vi "Visible_Ch.vi"(8 "Unit PN":string) -> ()   [LabVIEW 2017]
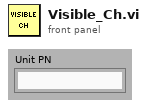
[diagram p1: front panel]
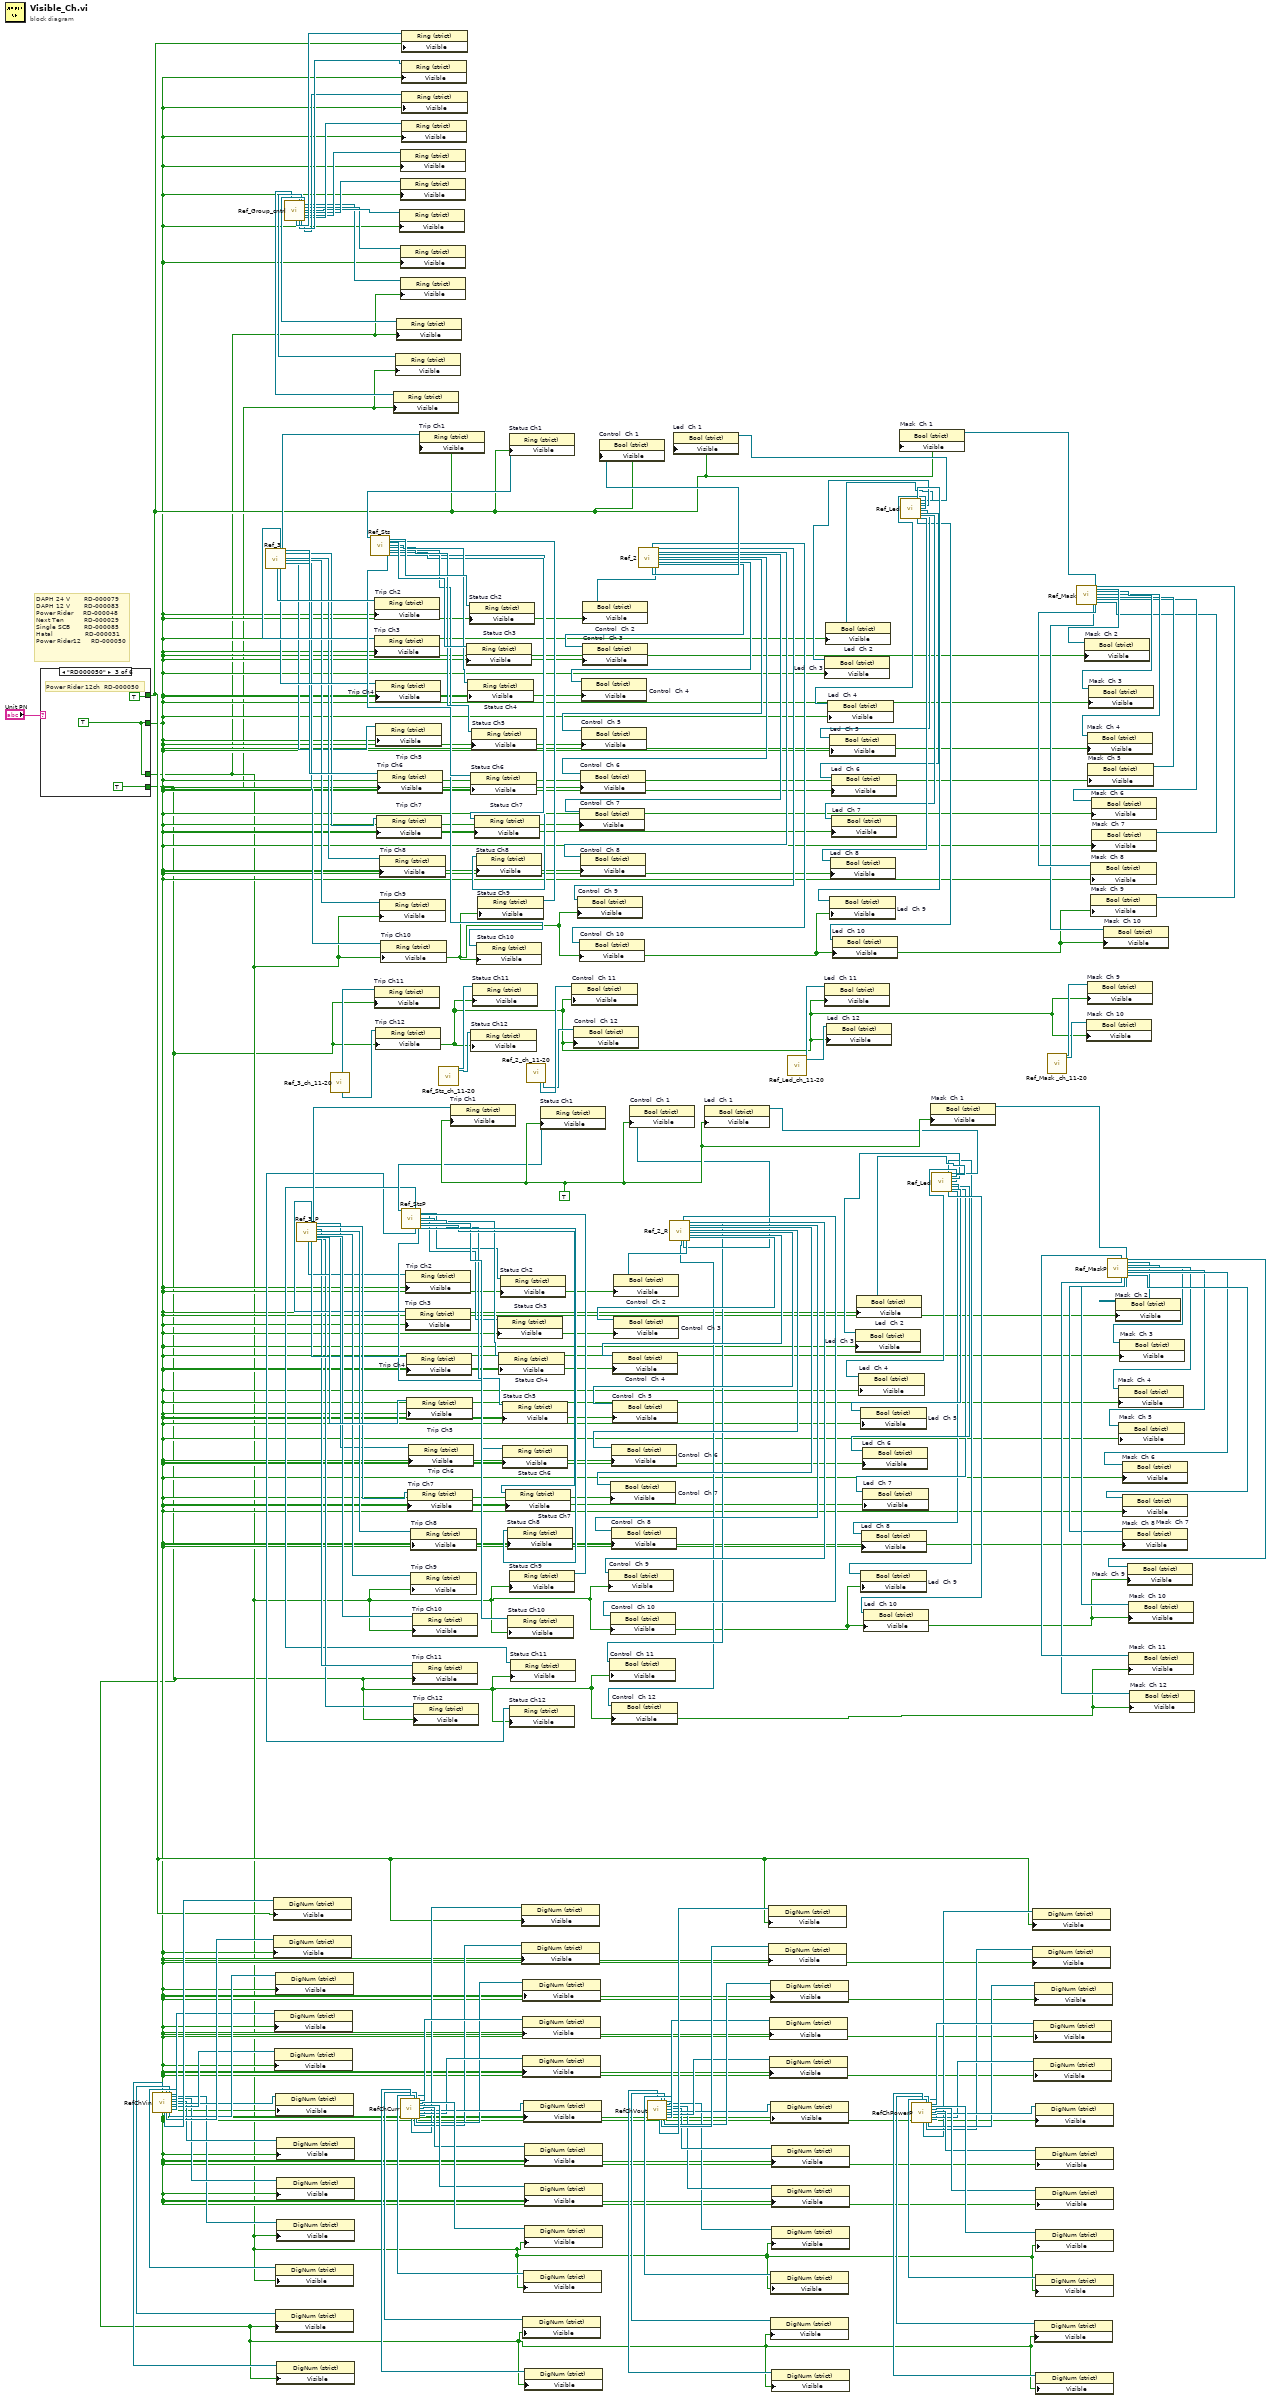
[diagram p0: block diagram]
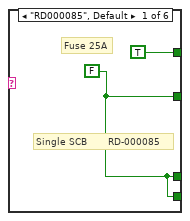
[diagram p2: hidden frame]
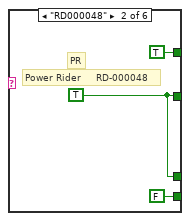
[diagram p3: hidden frame]
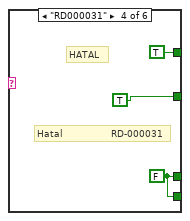
[diagram p4: hidden frame]
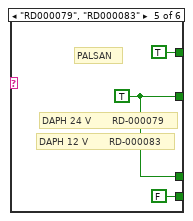
[diagram p5: hidden frame]
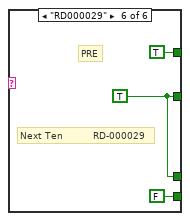
[diagram p6: hidden frame]
diagram:
  w133 = TRUE
  # "DAPH 24 V  \t    RD-000079\nDAPH 12 V  \t    RD-000083\nPower Rider \t   RD-000048\nNext Ten  \t       RD-000029\nSingle SCB       RD-000085 \nHatal                RD-000031\nPower Rider12 \t   RD-000050"
  n1 = case shown="\"RD000050\"" "Unit PN" {
    tunnel: [w186 w189 w192 TRUE w198 w201] -> w3
    tunnel: [w186 w189 w192 w194 w198 w201] -> w2
    tunnel: [w186 FALSE TRUE w194 FALSE FALSE] -> w1
    tunnel: [TRUE TRUE TRUE TRUE TRUE TRUE] -> w4
    frame "RD000085", Default {
      w186 = FALSE
      # "Single SCB       RD-000085"
      # "Fuse 25A"
    }
    frame "RD000048" {
      w189 = TRUE
      # "Power Rider \t   RD-000048"
      # "PR"
    }
    frame "RD000050" {
      w192 = TRUE
      # "Power Rider 12ch  RD-000050"
    }
    frame "RD000031" {
      w194 = FALSE
      # "Hatal                RD-000031"
      # "HATAL"
    }
    frame "RD000079", "RD000083" {
      w198 = TRUE
      # "DAPH 12 V  \t    RD-000083"
      # "DAPH 24 V  \t    RD-000079"
      # "PALSAN"
    }
    frame "RD000029" {
      w201 = TRUE
      # "Next Ten  \t       RD-000029"
      # "PRE"
    }
  }
  n2 = call "RefChVin.vi"() -> ("Vin  P1 out"=w64:refnum<vi>, "Vin  P12 out"=w53:refnum<vi>, "Vin  P2 out"=w63:refnum<vi>, "Vin  P11 out"=w54:refnum<vi>, "Vin  P3 out"=w62:refnum<vi>, "Vin  P10 out"=w55:refnum<vi>, "Vin  P9 out"=w56:refnum<vi>, "Vin  P8 out"=w57:refnum<vi>, "Vin  P7 out"=w58:refnum<vi>, "Vin  P6 out"=w59:refnum<vi>, "Vin  P5 out"=w60:refnum<vi>, "Vin  P4 out"=w61:refnum<vi>)  [unwired: 15 in, 1 out]
  n3 = call "Ref_3.vi"() -> ("Trip  Ch 1 out"=w184:refnum<vi>, "Trip  Ch 2 out"=w180:refnum<vi>, "Trip  Ch 3 out"=w164:refnum<vi>, "Trip  Ch 4 out"=w163:refnum<vi>, "Trip  Ch 5 out"=w144:refnum<vi>, "Trip  Ch 6 out"=w162:refnum<vi>, "Trip  Ch 7 out"=w161:refnum<vi>, "Trip  Ch 8 out"=w160:refnum<vi>, "Trip  Ch 9 out"=w159:refnum<vi>, "Trip  Ch 10 out"=w158:refnum<vi>)  [unwired: 18 in]
  n4 = property class="DigNum (strict)"(reference=w64, "Visible"=w4) -> ()  [unwired: 1 in, 2 out]
  n5 = property class="DigNum (strict)"(reference=w63, "Visible"=w3) -> ()  [unwired: 1 in, 2 out]
  n6 = property class="DigNum (strict)"(reference=w61, "Visible"=w3) -> ()  [unwired: 1 in, 2 out]
  n7 = property class="DigNum (strict)"(reference=w60, "Visible"=w3) -> ()  [unwired: 1 in, 2 out]
  n8 = property class="DigNum (strict)"(reference=w62, "Visible"=w3) -> ()  [unwired: 1 in, 2 out]
  n9 = property class="DigNum (strict)"(reference=w54, "Visible"=w1) -> ()  [unwired: 1 in, 2 out]
  n10 = property class="DigNum (strict)"(reference=w59, "Visible"=w3) -> ()  [unwired: 1 in, 2 out]
  n11 = property class="DigNum (strict)"(reference=w55, "Visible"=w2) -> ()  [unwired: 1 in, 2 out]
  n12 = property class="DigNum (strict)"(reference=w58, "Visible"=w3) -> ()  [unwired: 1 in, 2 out]
  n13 = property class="DigNum (strict)"(reference=w57, "Visible"=w3) -> ()  [unwired: 1 in, 2 out]
  n14 = property class="DigNum (strict)"(reference=w56, "Visible"=w2) -> ()  [unwired: 1 in, 2 out]
  n15 = property class="DigNum (strict)"(reference=w53, "Visible"=w1) -> ()  [unwired: 1 in, 2 out]
  n16 = call "Ref_Group_cntrl.vi"() -> ("Group ch 1 out"=w16:refnum<vi>, "Group ch 12 out"=w5:refnum<vi>, "Group ch 2 out"=w15:refnum<vi>, "Group ch 11 out"=w6:refnum<vi>, "Group ch 3 out"=w14:refnum<vi>, "Group ch 10 out"=w7:refnum<vi>, "Group ch 9 out"=w8:refnum<vi>, "Group ch 8 out"=w9:refnum<vi>, "Group ch 7 out"=w10:refnum<vi>, "Group ch 6 out"=w11:refnum<vi>, "Group ch 5 out"=w12:refnum<vi>, "Group ch 4 out"=w13:refnum<vi>)  [unwired: 15 in, 1 out]
  n17 = call "Ref_3_P.vi"() -> ("Trip  Ch 1 out"=w83:refnum<vi>, "Trip  Ch 2 out"=w86:refnum<vi>, "Trip  Ch 3 out"=w102:refnum<vi>, "Trip  Ch 4 out"=w103:refnum<vi>, "Trip  Ch 5 out"=w122:refnum<vi>, "Trip  Ch 6 out"=w104:refnum<vi>, "Trip  Ch 7 out"=w105:refnum<vi>, "Trip  Ch 11 out"=w82:refnum<vi>, "Trip  Ch 8 out"=w106:refnum<vi>, "Trip  Ch 9 out"=w107:refnum<vi>, "Trip  Ch 10 out"=w108:refnum<vi>, "Trip  Ch 12 out"=w81:refnum<vi>)  [unwired: 16 in]
  n18 = call "Ref_3_ch_11-20.vi"() -> ("Trip  Ch 11 out"=w68:refnum<vi>, "Trip  Ch 12 out"=w67:refnum<vi>)  [unwired: 18 in, 8 out]
  n19 = call "Ref_Sts.vi"() -> ("Status Ch9 out"=w166:refnum<vi>, "Status Ch10 out"=w165:refnum<vi>, "Status Ch1 out"=w183:refnum<vi>, "Status Ch2 out"=w172:refnum<vi>, "Status Ch3 out"=w171:refnum<vi>, "Status Ch4 out"=w170:refnum<vi>, "Status Ch5 out"=w169:refnum<vi>, "Status Ch6 out"=w168:refnum<vi>, "Status Ch7 out"=w167:refnum<vi>, "Status Ch8 out"=w155:refnum<vi>)  [unwired: 18 in]
  n20 = property on="Trip Ch3" class="Ring (strict)"(reference=w164, "Visible"=w3) -> ()  [unwired: 1 in, 2 out]
  n21 = property on="Trip Ch11" class="Ring (strict)"(reference=w68, "Visible"=w1) -> ()  [unwired: 1 in, 2 out]
  n22 = property on="Trip Ch2" class="Ring (strict)"(reference=w180, "Visible"=w3) -> ()  [unwired: 1 in, 2 out]
  n23 = property on="Trip Ch4" class="Ring (strict)"(reference=w163, "Visible"=w3) -> ()  [unwired: 1 in, 2 out]
  n24 = property on="Trip Ch12" class="Ring (strict)"(reference=w67, "Visible"=w1) -> ()  [unwired: 1 in, 2 out]
  n25 = property on="Trip Ch5" class="Ring (strict)"(reference=w144, "Visible"=w3) -> ()  [unwired: 1 in, 2 out]
  n26 = property on="Trip Ch7" class="Ring (strict)"(reference=w161, "Visible"=w3) -> ()  [unwired: 1 in, 2 out]
  n27 = property on="Trip Ch6" class="Ring (strict)"(reference=w162, "Visible"=w3) -> ()  [unwired: 1 in, 2 out]
  n28 = property on="Trip Ch8" class="Ring (strict)"(reference=w160, "Visible"=w3) -> ()  [unwired: 1 in, 2 out]
  n29 = property on="Trip Ch9" class="Ring (strict)"(reference=w159, "Visible"=w2) -> ()  [unwired: 1 in, 2 out]
  n30 = property on="Trip Ch10" class="Ring (strict)"(reference=w158, "Visible"=w2) -> ()  [unwired: 1 in, 2 out]
  n31 = property class="Ring (strict)"(reference=w5, "Visible"=w1) -> ()  [unwired: 1 in, 2 out]
  n32 = property class="Ring (strict)"(reference=w6, "Visible"=w1) -> ()  [unwired: 1 in, 2 out]
  n33 = property class="Ring (strict)"(reference=w7, "Visible"=w2) -> ()  [unwired: 1 in, 2 out]
  n34 = property class="Ring (strict)"(reference=w10, "Visible"=w3) -> ()  [unwired: 1 in, 2 out]
  n35 = property class="Ring (strict)"(reference=w12, "Visible"=w3) -> ()  [unwired: 1 in, 2 out]
  n36 = property class="Ring (strict)"(reference=w11, "Visible"=w3) -> ()  [unwired: 1 in, 2 out]
  n37 = property class="Ring (strict)"(reference=w9, "Visible"=w3) -> ()  [unwired: 1 in, 2 out]
  n38 = call "RefChCurr.vi"() -> ("Current P1 out"=w41:refnum<vi>, "Current P12 out"=w52:refnum<vi>, "Current P2 out"=w42:refnum<vi>, "Current P11 out"=w51:refnum<vi>, "Current P3 out"=w43:refnum<vi>, "Current P10 out"=w50:refnum<vi>, "Current P9 out"=w49:refnum<vi>, "Current P8 out"=w48:refnum<vi>, "Current P7 out"=w47:refnum<vi>, "Current P6 out"=w46:refnum<vi>, "Current P5 out"=w45:refnum<vi>, "Current P4 out"=w44:refnum<vi>)  [unwired: 15 in, 1 out]
  n39 = property class="Ring (strict)"(reference=w8, "Visible"=w2) -> ()  [unwired: 1 in, 2 out]
  n40 = property class="Ring (strict)"(reference=w15, "Visible"=w3) -> ()  [unwired: 1 in, 2 out]
  n41 = property class="Ring (strict)"(reference=w13, "Visible"=w3) -> ()  [unwired: 1 in, 2 out]
  n42 = call "Ref_StsP.vi"() -> ("Status Ch11 out"=w80:refnum<vi>, "Status Ch12 out"=w79:refnum<vi>, "Status Ch9 out"=w100:refnum<vi>, "Status Ch10 out"=w101:refnum<vi>, "Status Ch1 out"=w84:refnum<vi>, "Status Ch2 out"=w94:refnum<vi>, "Status Ch3 out"=w95:refnum<vi>, "Status Ch4 out"=w96:refnum<vi>, "Status Ch5 out"=w97:refnum<vi>, "Status Ch6 out"=w98:refnum<vi>, "Status Ch7 out"=w99:refnum<vi>, "Status Ch8 out"=w111:refnum<vi>)  [unwired: 16 in]
  n43 = property class="Ring (strict)"(reference=w16, "Visible"=w4) -> ()  [unwired: 1 in, 2 out]
  n44 = property class="Ring (strict)"(reference=w14, "Visible"=w3) -> ()  [unwired: 1 in, 2 out]
  n45 = property on="Trip Ch3" class="Ring (strict)"(reference=w102, "Visible"=w3) -> ()  [unwired: 1 in, 2 out]
  n46 = property on="Trip Ch2" class="Ring (strict)"(reference=w86, "Visible"=w3) -> ()  [unwired: 1 in, 2 out]
  n47 = property on="Trip Ch4" class="Ring (strict)"(reference=w103, "Visible"=w3) -> ()  [unwired: 1 in, 2 out]
  n48 = property on="Trip Ch5" class="Ring (strict)"(reference=w122, "Visible"=w3) -> ()  [unwired: 1 in, 2 out]
  n49 = property on="Trip Ch7" class="Ring (strict)"(reference=w105, "Visible"=w3) -> ()  [unwired: 1 in, 2 out]
  n50 = property on="Trip Ch6" class="Ring (strict)"(reference=w104, "Visible"=w3) -> ()  [unwired: 1 in, 2 out]
  n51 = property on="Trip Ch8" class="Ring (strict)"(reference=w106, "Visible"=w3) -> ()  [unwired: 1 in, 2 out]
  n52 = property on="Trip Ch9" class="Ring (strict)"(reference=w107, "Visible"=w2) -> ()  [unwired: 1 in, 2 out]
  n53 = property on="Trip Ch10" class="Ring (strict)"(reference=w108, "Visible"=w2) -> ()  [unwired: 1 in, 2 out]
  n54 = property on="Trip Ch11" class="Ring (strict)"(reference=w82, "Visible"=w1) -> ()  [unwired: 1 in, 2 out]
  n55 = property on="Trip Ch12" class="Ring (strict)"(reference=w81, "Visible"=w1) -> ()  [unwired: 1 in, 2 out]
  n56 = property on="Trip Ch1" class="Ring (strict)"(reference=w184, "Visible"=w4) -> ()  [unwired: 1 in, 2 out]
  n57 = call "Ref_Sts_ch_11-20.vi"() -> ("Status Ch 11 out"=w66:refnum<vi>, "Status Ch 12 out"=w65:refnum<vi>)  [unwired: 18 in, 8 out]
  n58 = property on="Trip Ch1" class="Ring (strict)"(reference=w83, "Visible"=w133) -> ()  [unwired: 1 in, 2 out]
  n59 = property on="Status Ch3" class="Ring (strict)"(reference=w171, "Visible"=w3) -> ()  [unwired: 1 in, 2 out]
  n60 = property on="Status Ch4" class="Ring (strict)"(reference=w170, "Visible"=w3) -> ()  [unwired: 1 in, 2 out]
  n61 = property on="Status Ch2" class="Ring (strict)"(reference=w172, "Visible"=w3) -> ()  [unwired: 1 in, 2 out]
  n62 = property on="Status Ch6" class="Ring (strict)"(reference=w168, "Visible"=w3) -> ()  [unwired: 1 in, 2 out]
  n63 = property on="Status Ch12" class="Ring (strict)"(reference=w65, "Visible"=w1) -> ()  [unwired: 1 in, 2 out]
  n64 = property on="Status Ch5" class="Ring (strict)"(reference=w169, "Visible"=w3) -> ()  [unwired: 1 in, 2 out]
  n65 = property on="Status Ch11" class="Ring (strict)"(reference=w66, "Visible"=w1) -> ()  [unwired: 1 in, 2 out]
  n66 = property on="Status Ch7" class="Ring (strict)"(reference=w167, "Visible"=w3) -> ()  [unwired: 1 in, 2 out]
  n67 = property on="Status Ch8" class="Ring (strict)"(reference=w155, "Visible"=w3) -> ()  [unwired: 1 in, 2 out]
  n68 = property on="Status Ch10" class="Ring (strict)"(reference=w165, "Visible"=w2) -> ()  [unwired: 1 in, 2 out]
  n69 = property on="Status Ch9" class="Ring (strict)"(reference=w166, "Visible"=w2) -> ()  [unwired: 1 in, 2 out]
  n70 = property on="Status Ch3" class="Ring (strict)"(reference=w95, "Visible"=w3) -> ()  [unwired: 1 in, 2 out]
  n71 = property on="Status Ch4" class="Ring (strict)"(reference=w96, "Visible"=w3) -> ()  [unwired: 1 in, 2 out]
  n72 = property on="Status Ch2" class="Ring (strict)"(reference=w94, "Visible"=w3) -> ()  [unwired: 1 in, 2 out]
  n73 = property on="Status Ch6" class="Ring (strict)"(reference=w98, "Visible"=w3) -> ()  [unwired: 1 in, 2 out]
  n74 = property on="Status Ch5" class="Ring (strict)"(reference=w97, "Visible"=w3) -> ()  [unwired: 1 in, 2 out]
  n75 = property on="Status Ch7" class="Ring (strict)"(reference=w99, "Visible"=w3) -> ()  [unwired: 1 in, 2 out]
  n76 = property on="Status Ch8" class="Ring (strict)"(reference=w111, "Visible"=w3) -> ()  [unwired: 1 in, 2 out]
  n77 = property on="Status Ch10" class="Ring (strict)"(reference=w101, "Visible"=w2) -> ()  [unwired: 1 in, 2 out]
  n78 = property on="Status Ch1" class="Ring (strict)"(reference=w183, "Visible"=w4) -> ()  [unwired: 1 in, 2 out]
  n79 = property on="Status Ch9" class="Ring (strict)"(reference=w100, "Visible"=w2) -> ()  [unwired: 1 in, 2 out]
  n80 = property on="Status Ch12" class="Ring (strict)"(reference=w79, "Visible"=w1) -> ()  [unwired: 1 in, 2 out]
  n81 = property on="Status Ch11" class="Ring (strict)"(reference=w80, "Visible"=w1) -> ()  [unwired: 1 in, 2 out]
  n82 = property class="DigNum (strict)"(reference=w41, "Visible"=w4) -> ()  [unwired: 1 in, 2 out]
  n83 = property class="DigNum (strict)"(reference=w42, "Visible"=w3) -> ()  [unwired: 1 in, 2 out]
  n84 = property class="DigNum (strict)"(reference=w44, "Visible"=w3) -> ()  [unwired: 1 in, 2 out]
  n85 = property class="DigNum (strict)"(reference=w45, "Visible"=w3) -> ()  [unwired: 1 in, 2 out]
  n86 = property class="DigNum (strict)"(reference=w43, "Visible"=w3) -> ()  [unwired: 1 in, 2 out]
  n87 = property class="DigNum (strict)"(reference=w51, "Visible"=w1) -> ()  [unwired: 1 in, 2 out]
  n88 = property class="DigNum (strict)"(reference=w46, "Visible"=w3) -> ()  [unwired: 1 in, 2 out]
  n89 = property class="DigNum (strict)"(reference=w50, "Visible"=w2) -> ()  [unwired: 1 in, 2 out]
  n90 = property class="DigNum (strict)"(reference=w47, "Visible"=w3) -> ()  [unwired: 1 in, 2 out]
  n91 = property class="DigNum (strict)"(reference=w48, "Visible"=w3) -> ()  [unwired: 1 in, 2 out]
  n92 = property class="DigNum (strict)"(reference=w49, "Visible"=w2) -> ()  [unwired: 1 in, 2 out]
  n93 = property class="DigNum (strict)"(reference=w52, "Visible"=w1) -> ()  [unwired: 1 in, 2 out]
  n94 = call "Ref_2_ch_11-20.vi"() -> ("Control  Ch 11 out"=w70:refnum<vi>, "Control  Ch 12 out"=w69:refnum<vi>)  [unwired: 17 in, 9 out]
  n95 = property on="Status Ch1" class="Ring (strict)"(reference=w84, "Visible"=w133) -> ()  [unwired: 1 in, 2 out]
  n96 = property on="Control  Ch 11" class="Bool (strict)"(reference=w70, "Visible"=w1) -> ()  [unwired: 1 in, 2 out]
  n97 = property on="Control  Ch 12" class="Bool (strict)"(reference=w69, "Visible"=w1) -> ()  [unwired: 1 in, 2 out]
  n98 = call "Ref_2.vi"() -> ("Control  Ch 10 out"=w173:refnum<vi>, "Control  Ch 1 out"=w182:refnum<vi>, "Control  Ch 9 out"=w174:refnum<vi>, "Control  Ch 2 out"=w179:refnum<vi>, "Control  Ch 8 out"=w175:refnum<vi>, "Control  Ch 7 out"=w176:refnum<vi>, "Control  Ch 6 out"=w156:refnum<vi>, "Control  Ch 5 out"=w177:refnum<vi>, "Control  Ch 4 out"=w178:refnum<vi>, "Control  Ch 3 out"=w157:refnum<vi>)  [unwired: 17 in, 1 out]
  n99 = property on="Control  Ch 9" class="Bool (strict)"(reference=w174, "Visible"=w2) -> ()  [unwired: 1 in, 2 out]
  n100 = property on="Control  Ch 7" class="Bool (strict)"(reference=w176, "Visible"=w3) -> ()  [unwired: 1 in, 2 out]
  n101 = property on="Control  Ch 10" class="Bool (strict)"(reference=w173, "Visible"=w2) -> ()  [unwired: 1 in, 2 out]
  n102 = property on="Control  Ch 6" class="Bool (strict)"(reference=w156, "Visible"=w3) -> ()  [unwired: 1 in, 2 out]
  n103 = property on="Control  Ch 8" class="Bool (strict)"(reference=w175, "Visible"=w3) -> ()  [unwired: 1 in, 2 out]
  n104 = property on="Control  Ch 4" class="Bool (strict)"(reference=w178, "Visible"=w3) -> ()  [unwired: 1 in, 2 out]
  n105 = property on="Control  Ch 5" class="Bool (strict)"(reference=w177, "Visible"=w3) -> ()  [unwired: 1 in, 2 out]
  n106 = property on="Control  Ch 2" class="Bool (strict)"(reference=w179, "Visible"=w3) -> ()  [unwired: 1 in, 2 out]
  n107 = property on="Control  Ch 3" class="Bool (strict)"(reference=w157, "Visible"=w3) -> ()  [unwired: 1 in, 2 out]
  n108 = property on="Control  Ch 1" class="Bool (strict)"(reference=w182, "Visible"=w4) -> ()  [unwired: 1 in, 2 out]
  n109 = call "RefChVout.vi"() -> ("Vout  P1 out"=w40:refnum<vi>, "Vout  P12 out"=w29:refnum<vi>, "Vout  P2 out"=w39:refnum<vi>, "Vout  P11 out"=w30:refnum<vi>, "Vout  P3 out"=w38:refnum<vi>, "Vout  P10 out"=w31:refnum<vi>, "Vout  P9 out"=w32:refnum<vi>, "Vout  P8 out"=w33:refnum<vi>, "Vout  P7 out"=w34:refnum<vi>, "Vout  P6 out"=w35:refnum<vi>, "Vout  P5 out"=w36:refnum<vi>, "Vout  P4 out"=w37:refnum<vi>)  [unwired: 15 in, 1 out]
  n110 = call "Ref_2_R.vi"() -> ("Control  Ch 12 out"=w77:refnum<vi>, "Control  Ch 10 out"=w93:refnum<vi>, "Control  Ch 1 out"=w85:refnum<vi>, "Control  Ch 9 out"=w92:refnum<vi>, "Control  Ch 2 out"=w87:refnum<vi>, "Control  Ch 11 out"=w78:refnum<vi>, "Control  Ch 8 out"=w91:refnum<vi>, "Control  Ch 7 out"=w90:refnum<vi>, "Control  Ch 6 out"=w110:refnum<vi>, "Control  Ch 5 out"=w89:refnum<vi>, "Control  Ch 4 out"=w88:refnum<vi>, "Control  Ch 3 out"=w109:refnum<vi>)  [unwired: 15 in, 1 out]
  n111 = property on="Control  Ch 9" class="Bool (strict)"(reference=w92, "Visible"=w2) -> ()  [unwired: 1 in, 2 out]
  n112 = property on="Control  Ch 11" class="Bool (strict)"(reference=w78, "Visible"=w1) -> ()  [unwired: 1 in, 2 out]
  n113 = property on="Control  Ch 7" class="Bool (strict)"(reference=w90, "Visible"=w3) -> ()  [unwired: 1 in, 2 out]
  n114 = property on="Control  Ch 10" class="Bool (strict)"(reference=w93, "Visible"=w2) -> ()  [unwired: 1 in, 2 out]
  n115 = property on="Control  Ch 6" class="Bool (strict)"(reference=w110, "Visible"=w3) -> ()  [unwired: 1 in, 2 out]
  n116 = property on="Control  Ch 8" class="Bool (strict)"(reference=w91, "Visible"=w3) -> ()  [unwired: 1 in, 2 out]
  n117 = property on="Control  Ch 12" class="Bool (strict)"(reference=w77, "Visible"=w1) -> ()  [unwired: 1 in, 2 out]
  n118 = property on="Control  Ch 4" class="Bool (strict)"(reference=w88, "Visible"=w3) -> ()  [unwired: 1 in, 2 out]
  n119 = property on="Control  Ch 5" class="Bool (strict)"(reference=w89, "Visible"=w3) -> ()  [unwired: 1 in, 2 out]
  n120 = property on="Control  Ch 2" class="Bool (strict)"(reference=w87, "Visible"=w3) -> ()  [unwired: 1 in, 2 out]
  n121 = property on="Control  Ch 3" class="Bool (strict)"(reference=w109, "Visible"=w3) -> ()  [unwired: 1 in, 2 out]
  n122 = property on="Control  Ch 1" class="Bool (strict)"(reference=w85, "Visible"=w133) -> ()  [unwired: 1 in, 2 out]
  n123 = property class="DigNum (strict)"(reference=w40, "Visible"=w4) -> ()  [unwired: 1 in, 2 out]
  n124 = property class="DigNum (strict)"(reference=w39, "Visible"=w3) -> ()  [unwired: 1 in, 2 out]
  n125 = property class="DigNum (strict)"(reference=w37, "Visible"=w3) -> ()  [unwired: 1 in, 2 out]
  n126 = property class="DigNum (strict)"(reference=w36, "Visible"=w3) -> ()  [unwired: 1 in, 2 out]
  n127 = property class="DigNum (strict)"(reference=w38, "Visible"=w3) -> ()  [unwired: 1 in, 2 out]
  n128 = property class="DigNum (strict)"(reference=w30, "Visible"=w1) -> ()  [unwired: 1 in, 2 out]
  n129 = property class="DigNum (strict)"(reference=w35, "Visible"=w3) -> ()  [unwired: 1 in, 2 out]
  n130 = property class="DigNum (strict)"(reference=w31, "Visible"=w2) -> ()  [unwired: 1 in, 2 out]
  n131 = property class="DigNum (strict)"(reference=w34, "Visible"=w3) -> ()  [unwired: 1 in, 2 out]
  n132 = property class="DigNum (strict)"(reference=w33, "Visible"=w3) -> ()  [unwired: 1 in, 2 out]
  n133 = property class="DigNum (strict)"(reference=w32, "Visible"=w2) -> ()  [unwired: 1 in, 2 out]
  n134 = property class="DigNum (strict)"(reference=w29, "Visible"=w1) -> ()  [unwired: 1 in, 2 out]
  n135 = call "Ref_Led_ch_11-20.vi"() -> ("Led Ch 11 out"=w72:refnum<vi>, "Led Ch 12 out"=w71:refnum<vi>)  [unwired: 18 in, 8 out]
  n136 = property on="Led  Ch 11" class="Bool (strict)"(reference=w72, "Visible"=w1) -> ()  [unwired: 1 in, 2 out]
  n137 = property on="Led  Ch 12" class="Bool (strict)"(reference=w71, "Visible"=w1) -> ()  [unwired: 1 in, 2 out]
  n138 = call "Ref_Led.vi"() -> ("Led Ch 9 out"=w154:refnum<vi>, "Led Ch 10 out"=w147:refnum<vi>, "Led Ch 1 out"=w146:refnum<vi>, "Led Ch 2 out"=w145:refnum<vi>, "Led Ch 3 out"=w148:refnum<vi>, "Led Ch 4 out"=w149:refnum<vi>, "Led Ch 5 out"=w150:refnum<vi>, "Led Ch 6 out"=w151:refnum<vi>, "Led Ch 7 out"=w152:refnum<vi>, "Led Ch 8 out"=w153:refnum<vi>)  [unwired: 18 in]
  n139 = property on="Led  Ch 1" class="Bool (strict)"(reference=w146, "Visible"=w4) -> ()  [unwired: 1 in, 2 out]
  n140 = property on="Led  Ch 3" class="Bool (strict)"(reference=w148, "Visible"=w3) -> ()  [unwired: 1 in, 2 out]
  n141 = property on="Led  Ch 2" class="Bool (strict)"(reference=w145, "Visible"=w3) -> ()  [unwired: 1 in, 2 out]
  n142 = property on="Led  Ch 4" class="Bool (strict)"(reference=w149, "Visible"=w3) -> ()  [unwired: 1 in, 2 out]
  n143 = property on="Led  Ch 5" class="Bool (strict)"(reference=w150, "Visible"=w3) -> ()  [unwired: 1 in, 2 out]
  n144 = property on="Led  Ch 9" class="Bool (strict)"(reference=w154, "Visible"=w2) -> ()  [unwired: 1 in, 2 out]
  n145 = property on="Led  Ch 8" class="Bool (strict)"(reference=w153, "Visible"=w3) -> ()  [unwired: 1 in, 2 out]
  n146 = property on="Led  Ch 6" class="Bool (strict)"(reference=w151, "Visible"=w3) -> ()  [unwired: 1 in, 2 out]
  n147 = property on="Led  Ch 7" class="Bool (strict)"(reference=w152, "Visible"=w3) -> ()  [unwired: 1 in, 2 out]
  n148 = property on="Led  Ch 10" class="Bool (strict)"(reference=w147, "Visible"=w2) -> ()  [unwired: 1 in, 2 out]
  n149 = call "RefChPowerP.vi"() -> ("Pwr  P1 out"=w17:refnum<vi>, "Pwr  P12 out"=w28:refnum<vi>, "Pwr  P2 out"=w18:refnum<vi>, "Pwr  P11 out"=w27:refnum<vi>, "Pwr  P3 out"=w19:refnum<vi>, "Pwr  P10 out"=w26:refnum<vi>, "Pwr  P9 out"=w25:refnum<vi>, "Pwr  P8 out"=w24:refnum<vi>, "Pwr  P7 out"=w23:refnum<vi>, "Pwr  P6 out"=w22:refnum<vi>, "Pwr  P5 out"=w21:refnum<vi>, "Pwr  P4 out"=w20:refnum<vi>)  [unwired: 15 in, 1 out]
  n150 = call "Ref_Led.vi"() -> ("Led Ch 9 out"=w112:refnum<vi>, "Led Ch 10 out"=w119:refnum<vi>, "Led Ch 1 out"=w120:refnum<vi>, "Led Ch 2 out"=w121:refnum<vi>, "Led Ch 3 out"=w118:refnum<vi>, "Led Ch 4 out"=w117:refnum<vi>, "Led Ch 5 out"=w116:refnum<vi>, "Led Ch 6 out"=w115:refnum<vi>, "Led Ch 7 out"=w114:refnum<vi>, "Led Ch 8 out"=w113:refnum<vi>)  [unwired: 18 in]
  n151 = property on="Led  Ch 1" class="Bool (strict)"(reference=w120, "Visible"=w133) -> ()  [unwired: 1 in, 2 out]
  n152 = property on="Led  Ch 3" class="Bool (strict)"(reference=w118, "Visible"=w3) -> ()  [unwired: 1 in, 2 out]
  n153 = property on="Led  Ch 2" class="Bool (strict)"(reference=w121, "Visible"=w3) -> ()  [unwired: 1 in, 2 out]
  n154 = property on="Led  Ch 4" class="Bool (strict)"(reference=w117, "Visible"=w3) -> ()  [unwired: 1 in, 2 out]
  n155 = property on="Led  Ch 5" class="Bool (strict)"(reference=w116, "Visible"=w3) -> ()  [unwired: 1 in, 2 out]
  n156 = property on="Led  Ch 9" class="Bool (strict)"(reference=w112, "Visible"=w2) -> ()  [unwired: 1 in, 2 out]
  n157 = property on="Led  Ch 8" class="Bool (strict)"(reference=w113, "Visible"=w3) -> ()  [unwired: 1 in, 2 out]
  n158 = property on="Led  Ch 6" class="Bool (strict)"(reference=w115, "Visible"=w3) -> ()  [unwired: 1 in, 2 out]
  n159 = property on="Led  Ch 7" class="Bool (strict)"(reference=w114, "Visible"=w3) -> ()  [unwired: 1 in, 2 out]
  n160 = property on="Led  Ch 10" class="Bool (strict)"(reference=w119, "Visible"=w2) -> ()  [unwired: 1 in, 2 out]
  n161 = property class="DigNum (strict)"(reference=w17, "Visible"=w4) -> ()  [unwired: 1 in, 2 out]
  n162 = property class="DigNum (strict)"(reference=w18, "Visible"=w3) -> ()  [unwired: 1 in, 2 out]
  n163 = property class="DigNum (strict)"(reference=w20, "Visible"=w3) -> ()  [unwired: 1 in, 2 out]
  n164 = property class="DigNum (strict)"(reference=w21, "Visible"=w3) -> ()  [unwired: 1 in, 2 out]
  n165 = property class="DigNum (strict)"(reference=w19, "Visible"=w3) -> ()  [unwired: 1 in, 2 out]
  n166 = property class="DigNum (strict)"(reference=w27, "Visible"=w1) -> ()  [unwired: 1 in, 2 out]
  n167 = property class="DigNum (strict)"(reference=w22, "Visible"=w3) -> ()  [unwired: 1 in, 2 out]
  n168 = property class="DigNum (strict)"(reference=w26, "Visible"=w2) -> ()  [unwired: 1 in, 2 out]
  n169 = property class="DigNum (strict)"(reference=w23, "Visible"=w3) -> ()  [unwired: 1 in, 2 out]
  n170 = property class="DigNum (strict)"(reference=w24, "Visible"=w3) -> ()  [unwired: 1 in, 2 out]
  n171 = property class="DigNum (strict)"(reference=w25, "Visible"=w2) -> ()  [unwired: 1 in, 2 out]
  n172 = property class="DigNum (strict)"(reference=w28, "Visible"=w1) -> ()  [unwired: 1 in, 2 out]
  n173 = call "Ref_Mask _ch_11-20.vi"() -> ("Mask Ch 11 out"=w73:refnum<vi>, "Mask Ch 12 out"=w74:refnum<vi>)  [unwired: 18 in, 8 out]
  n174 = call "Ref_Mask.vi"() -> ("Mask Ch 9 out"=w134:refnum<vi>, "Mask Ch 10 out"=w136:refnum<vi>, "Mask Ch 1 out"=w135:refnum<vi>, "Mask Ch 2 out"=w143:refnum<vi>, "Mask Ch 3 out"=w142:refnum<vi>, "Mask Ch 4 out"=w141:refnum<vi>, "Mask Ch 5 out"=w140:refnum<vi>, "Mask Ch 6 out"=w139:refnum<vi>, "Mask Ch 7 out"=w138:refnum<vi>, "Mask Ch 8 out"=w137:refnum<vi>)  [unwired: 18 in]
  n175 = property on="Mask  Ch 1" class="Bool (strict)"(reference=w135, "Visible"=w4) -> ()  [unwired: 1 in, 2 out]
  n176 = property on="Mask  Ch 2" class="Bool (strict)"(reference=w143, "Visible"=w3) -> ()  [unwired: 1 in, 2 out]
  n177 = property on="Mask  Ch 10" class="Bool (strict)"(reference=w74, "Visible"=w1) -> ()  [unwired: 1 in, 2 out]
  n178 = property on="Mask  Ch 4" class="Bool (strict)"(reference=w141, "Visible"=w3) -> ()  [unwired: 1 in, 2 out]
  n179 = property on="Mask  Ch 9" class="Bool (strict)"(reference=w73, "Visible"=w1) -> ()  [unwired: 1 in, 2 out]
  n180 = property on="Mask  Ch 5" class="Bool (strict)"(reference=w140, "Visible"=w3) -> ()  [unwired: 1 in, 2 out]
  n181 = property on="Mask  Ch 3" class="Bool (strict)"(reference=w142, "Visible"=w3) -> ()  [unwired: 1 in, 2 out]
  n182 = property on="Mask  Ch 8" class="Bool (strict)"(reference=w137, "Visible"=w3) -> ()  [unwired: 1 in, 2 out]
  n183 = property on="Mask  Ch 9" class="Bool (strict)"(reference=w134, "Visible"=w2) -> ()  [unwired: 1 in, 2 out]
  n184 = property on="Mask  Ch 6" class="Bool (strict)"(reference=w139, "Visible"=w3) -> ()  [unwired: 1 in, 2 out]
  n185 = property on="Mask  Ch 7" class="Bool (strict)"(reference=w138, "Visible"=w3) -> ()  [unwired: 1 in, 2 out]
  n186 = property on="Mask  Ch 10" class="Bool (strict)"(reference=w136, "Visible"=w2) -> ()  [unwired: 1 in, 2 out]
  n187 = call "Ref_MaskP.vi"() -> ("Mask Ch 11 out"=w76:refnum<vi>, "Mask Ch 12 out"=w75:refnum<vi>, "Mask Ch 9 out"=w132:refnum<vi>, "Mask Ch 10 out"=w130:refnum<vi>, "Mask Ch 1 out"=w131:refnum<vi>, "Mask Ch 2 out"=w123:refnum<vi>, "Mask Ch 3 out"=w124:refnum<vi>, "Mask Ch 4 out"=w125:refnum<vi>, "Mask Ch 5 out"=w126:refnum<vi>, "Mask Ch 6 out"=w127:refnum<vi>, "Mask Ch 7 out"=w128:refnum<vi>, "Mask Ch 8 out"=w129:refnum<vi>)  [unwired: 16 in]
  n188 = property on="Mask  Ch 1" class="Bool (strict)"(reference=w131, "Visible"=w133) -> ()  [unwired: 1 in, 2 out]
  n189 = property on="Mask  Ch 2" class="Bool (strict)"(reference=w123, "Visible"=w3) -> ()  [unwired: 1 in, 2 out]
  n190 = property on="Mask  Ch 4" class="Bool (strict)"(reference=w125, "Visible"=w3) -> ()  [unwired: 1 in, 2 out]
  n191 = property on="Mask  Ch 5" class="Bool (strict)"(reference=w126, "Visible"=w3) -> ()  [unwired: 1 in, 2 out]
  n192 = property on="Mask  Ch 3" class="Bool (strict)"(reference=w124, "Visible"=w3) -> ()  [unwired: 1 in, 2 out]
  n193 = property on="Mask  Ch 8" class="Bool (strict)"(reference=w129, "Visible"=w3) -> ()  [unwired: 1 in, 2 out]
  n194 = property on="Mask  Ch 6" class="Bool (strict)"(reference=w127, "Visible"=w3) -> ()  [unwired: 1 in, 2 out]
  n195 = property on="Mask  Ch 7" class="Bool (strict)"(reference=w128, "Visible"=w3) -> ()  [unwired: 1 in, 2 out]
  n196 = property on="Mask  Ch 9" class="Bool (strict)"(reference=w132, "Visible"=w2) -> ()  [unwired: 1 in, 2 out]
  n197 = property on="Mask  Ch 10" class="Bool (strict)"(reference=w130, "Visible"=w2) -> ()  [unwired: 1 in, 2 out]
  n198 = property on="Mask  Ch 11" class="Bool (strict)"(reference=w76, "Visible"=w1) -> ()  [unwired: 1 in, 2 out]
  n199 = property on="Mask  Ch 12" class="Bool (strict)"(reference=w75, "Visible"=w1) -> ()  [unwired: 1 in, 2 out]
